vi "set_lines_per_frame.vi"(8 "error in (no error)":errorcluster, 11 "ScanModeCN090721ThreeDScan in":refnum<class "ImagingModeDL100901FlexTrajectory.lvclass">) -> (0 "error out":errorcluster, 3 "ScanModeCN090721ThreeDScan out":refnum<class "ImagingModeDL100901FlexTrajectory.lvclass">)   [LabVIEW 2010, in "ImagingModeDL100901FlexTrajectory.lvclass"]
uses:
  ImagingModeDL100901FlexTrajectory.lvclass
  ImagingModeDL100901FlexTrajectory.lvclass/ImagingModeDL100901FlexTrajectory.ctl
panel:
  in  "lines per frame":i32
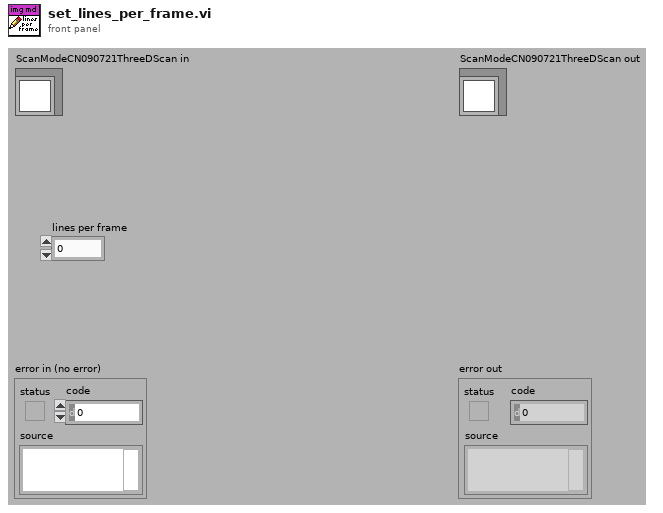
[diagram p1: front panel]
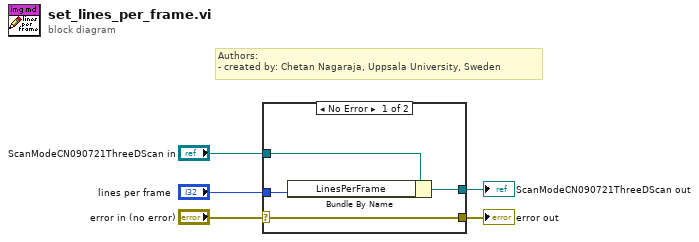
[diagram p0: block diagram]
diagram:
  # "Authors: \n- created by: Chetan Nagaraja, Uppsala University, Sweden"
  n1 = case shown="No Error" "error in (no error)" {
    selector: "error in (no error)" -> [w9 w11]
    tunnel: [w9 w11] -> w4
    tunnel: [w6 w10] -> w2
    tunnel: "ScanModeCN090721ThreeDScan in" -> [w7 w10]
    tunnel: "lines per frame" -> [w8 _]
    frame No Error {
      n2 = Bundle By Name(cluster=w7, "LinesPerFrame"=w8) -> (w6:refnum<class "ImagingModeDL100901FlexTrajectory.lvclass">)
    }
    frame Error {
    }
  }
  "error out" <- w4
  "ScanModeCN090721ThreeDScan out" <- w2
